vi "slopeAndIntercept.vi"() -> (0 "New Values In":string[][](array[string]), 1 "New Chs In":string[](array[string]))   [LabVIEW 2022 SP3]
uses:
  <vilib>/Analysis/6fits.llb/Curve Fitting Criteria.ctl
  Data plotting/subVIs/Plot_Values_Global.vi
  Results_plotter_Global.vi
  <vilib>/Analysis/NI_AALPro.lvlib
panel:
  in  "method":T1 items=["Least Square", "Least Absolute Residual", "Bisquare"]
  # "This VI calculates the slope and intercept of the series passed to it, and injects the values back to the results file."
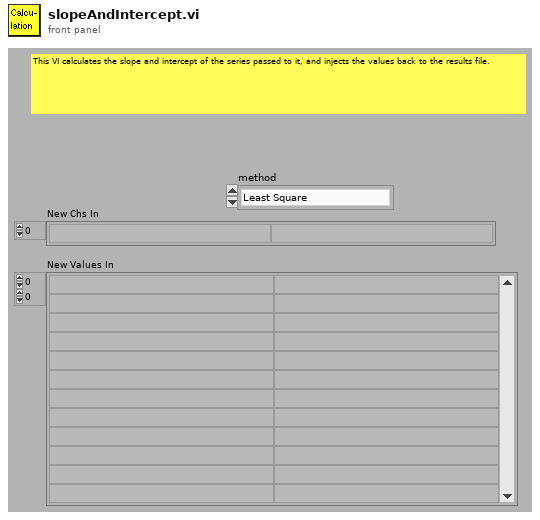
[diagram p1: front panel]
types:
  T1 = typedef "NI_AALPro.lvlib/Curve Fitting Criteria.ctl" = u16
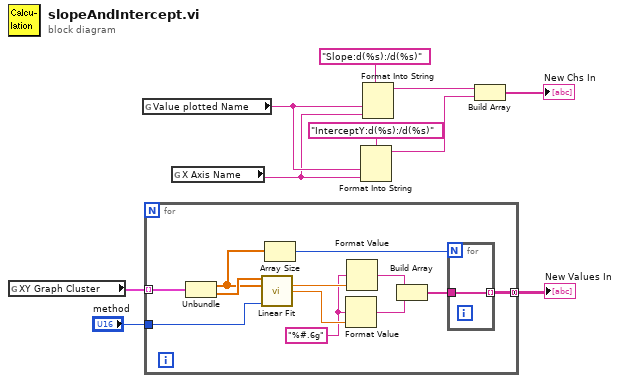
[diagram p0: block diagram]
diagram:
  n1 = global read "Plot_Values_Global.vi" "XY Graph Cluster"() -> (w9:cluster{dbl[], dbl[]}[])
  n2 = global read "Results_plotter_Global.vi" "Value plotted Name"() -> (w4:string)
  n3 = for {
    tunnel: w9 -> [w22] mode=indexing
    tunnel: "method" -> [w21]
    tunnel: [w11] -> w1 mode=concatenating
    w18 = "%#.6g" ("format string")
    n4 = Unbundle(w22) -> (w12:dbl[], w14:dbl[])
    n5 = call <vilib>:"Linear Fit.vi"("Y"=w14, "X"=w12, "method"=w21) -> ("slope"=w20:dbl, "intercept"=w19:dbl)  [unwired: 8 in, 3 out]
    n6 = Array Size(array=w12) -> (size(s)=w13:i32)
    n7 = Format Value(format string=w18, value (0)=w19) -> (output string=w16:string)  [unwired: 1 in]
    n8 = Format Value(format string=w18, value (0)=w20) -> (output string=w17:string)  [unwired: 1 in]
    n9 = Build Array(w17, w16) -> (w15:string[])
    n10 = for {
      N: w13 -> [_]
      tunnel: w15 -> [w23]
      tunnel: [w23] -> w11 mode=indexing
    }
  }
  "New Values In" <- w1
  n11 = global read "Results_plotter_Global.vi" "X Axis Name"() -> (w3:string)
  n12 = Format Into String(format string="InterceptY:d(%s):/d(%s)", w4, w3) -> (resulting string=w8:string)  [unwired: 2 in, 1 out]
  n13 = Format Into String(format string="Slope:d(%s):/d(%s)" ("string"), w4, w3) -> (resulting string=w7:string)  [unwired: 2 in, 1 out]
  n14 = Build Array(w7, w8) -> (→"New Chs In":string[])
